vi "GT Get Interrupt Time Max.vi"(8 "error in (no error)":errorcluster caption="错误输入（无错误）", 9 "pProfileRunTimeMax":dbl, 10 "pServoRunTimeMax":dbl, 11 "cardNum":i16) -> (0 "error out":errorcluster caption="错误输出", 1 "pProfileRunTimeMax out":dbl, 2 "pServoRunTimeMax out":dbl, 3 "function return":i16)   [LabVIEW 2020, in "gts1.lvlib"]
doc: "GT_API GT_GetInterruptTimeMax(short cardNum,double *pServoRunTimeMax,double *pProfileRunTimeMax);"
uses:
  gts1.lvlib
  dll/32bit/multi_card/gts.dll
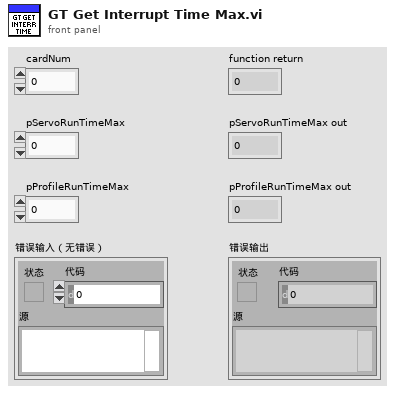
[diagram p1: front panel]
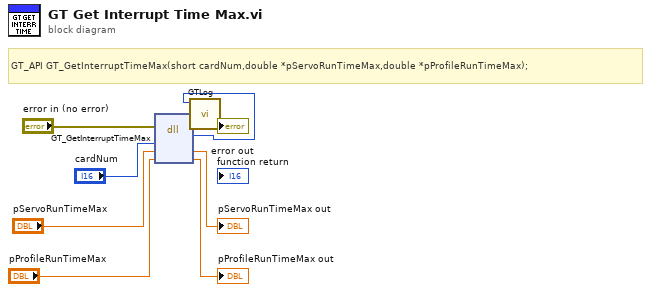
[diagram p0: block diagram]
diagram:
  # "GT_API GT_GetInterruptTimeMax(short cardNum,double *pServoRunTimeMax,double *pProfileRunTimeMax);"
  n1 = dll-call lib="C:/1228/dll/32bit/multi_card/gts.dll" fn="GT_GetInterruptTimeMax"(error in="error in (no error)", "cardNum"="cardNum", "pServoRunTimeMax"="pServoRunTimeMax", "pProfileRunTimeMax"="pProfileRunTimeMax") -> (error out=w3:errorcluster, w1:i16, "pServoRunTimeMax"=→"pServoRunTimeMax out":dbl, "pProfileRunTimeMax"=→"pProfileRunTimeMax out":dbl)  [unwired: 3 in, 1 out]
  n2 = call "GTLog.vi"("error in (no error)"=w3, "Numeric"=w1) -> ("error out"=→"error out":errorcluster)  [unwired: 9 in]
